vi "Test Threaded Parallel.vi"() -> ()   [LabVIEW 2021]
uses:
  Source/Support/Nodes/abs_Node/Status.ctl
  Test System/Test System.lvclass
  C:/Users/Tim/Documents/GitHub/LV_Behaviour_Tree/Source/System/bt_System.lvclass
  Source/Blackboard/Blackboard.lvclass
  Source/Support/Nodes/Decorators/Repeater/Support/Finish On - Type.ctl
  Source/Blackboard/Blackboard.lvclass/Blackboard.ctl
  Source/Support/Nodes/Leaves/abs_Type Leaf/abs_Type Leaf.lvclass/abs_Type Leaf.ctl
  Source/Support/Nodes/Composites/abs_Parallel/Support/Status Calculation.ctl
  Source/System/bt_System.lvclass/bt_System.ctl
  Source/Blackboard/Get Value Type/Get I32.vi
  <vilib>/TSA/Abstract Data Classes/Abs_Types/I32 Integer/Static Read.vi
  Source/System/Properties/Write Behaviour Tree.vi
  Source/Blackboard/Support/Index Group.vi
  Source/Blackboard/Support/Index Tags.vi
  Source/Support/Nodes/Leaves/abs_Type Leaf/Properties/Write Value Class.vi
  <vilib>/TSA/Omni-Bus/Local Bus/Support/I32/Local Bus_I32.lvclass
  C:/Program Files (x86)/National Instruments/LabVIEW 2021/vi.lib/TSA/Abstract Data Classes/Abs_Types/Value/Abs_Value.lvclass
  <vilib>/TSA/Abstract Data Classes/Abs_Types/I32 Integer/Abs_I32 Integer.lvclass
  C:/Program Files (x86)/National Instruments/LabVIEW 2021/vi.lib/TSA/Abstract Data Classes/Abs_Types/Numeric/Abs_Numeric.lvclass
  Source/Support/Nodes/Leaves/Test Boolean/Test Abs_Boolean.lvclass
  C:/Users/Tim/Documents/GitHub/LV_Behaviour_Tree/Source/Support/Nodes/abs_Node/bt_Node.lvclass
  C:/Users/Tim/Documents/GitHub/LV_Behaviour_Tree/BT Abstract Type/abs_Type Leaf/abs_Type Leaf.lvclass
  <vilib>/TSA/Abstract Data Classes/Abs_Types/Boolean/Abs_Boolean.lvclass
  C:/Program Files (x86)/National Instruments/LabVIEW 2021/vi.lib/TSA/Abstract Data Classes/Abs_Types/Type/Abs_Type.lvclass
  <vilib>/TSA/Omni-Bus/Local Bus/Support/Initialise DVR's.vi
  <vilib>/TSA/Abstract Data Classes/Functions/Math/Support/Increment/I32/Method.vi
  <vilib>/TSA/Abstract Data Classes/Constants/Support/I32/I32.vi
  <vilib>/TSA/Abstract Data Classes/Functions/Math/Support/Add/I32/Method.vi
  <vilib>/TSA/Abstract Data Classes/Functions/Compare/Support/Less/I32/Method.vi
  <vilib>/TSA/Abstract Data Classes/Abs_Types/Value/Abs_Value.lvclass
  <vilib>/TSA/Abstract Data Classes/Abs_Types/Type/Abs_Type.lvclass
  <vilib>/TSA/Omni-Bus/Local Bus/Support/DBL/Local Bus_DBL.lvclass
  <vilib>/TSA/Omni-Bus/Local Bus/Support/SGL/Local Bus_SGL.lvclass
  <vilib>/TSA/Omni-Bus/Local Bus/Support/EXT/Local Bus_EXT.lvclass
  <vilib>/TSA/Omni-Bus/Local Bus/Support/Bool/Local Bus_Boolean.lvclass
  <vilib>/TSA/Omni-Bus/Local Bus/Support/STR/Local Bus_String.lvclass
  <vilib>/TSA/Omni-Bus/Local Bus/Support/Variant/Local Bus_Variant.lvclass
  <vilib>/TSA/Omni-Bus/Local Bus/Support/WFM/Local Bus_Waveform.lvclass
  <vilib>/TSA/Omni-Bus/Local Bus/Support/Time/Local Bus_Time.lvclass
  <vilib>/TSA/Omni-Bus/Local Bus/Support/U8/Local Bus_U8.lvclass
  <vilib>/TSA/Omni-Bus/Local Bus/Support/U16/Local Bus_U16.lvclass
  <vilib>/TSA/Omni-Bus/Local Bus/Support/U32/Local Bus_U32.lvclass
  <vilib>/TSA/Omni-Bus/Local Bus/Support/U64/Local Bus_U64.lvclass
  <vilib>/TSA/Omni-Bus/Local Bus/Support/I8/Local Bus_I8.lvclass
  <vilib>/TSA/Omni-Bus/Local Bus/Support/I16/Local Bus_I16.lvclass
  <vilib>/TSA/Omni-Bus/Local Bus/Support/I64/Local Bus_I64.lvclass
  <vilib>/TSA/Omni-Bus/Local Bus/Support/CSGL/Local Bus_CSGL.lvclass
  <vilib>/TSA/Omni-Bus/Local Bus/Support/CDBL/Local Bus_CDBL.lvclass
  <vilib>/TSA/Omni-Bus/Local Bus/Support/CEXT/Local Bus_CEXT.lvclass
  Source/BT.lvlib
  Source/Support/Nodes/Decorators/Repeater/bt_Repeater.lvclass
  Source/System/bt_System.lvclass
  Source/Support/Nodes/Composites/abs_Parallel/bt_Parallel.lvclass
  C:/Program Files (x86)/National Instruments/LabVIEW 2021/vi.lib/TSA/Abstract Data Classes/Abs_Types/Integer/Abs_Integer.lvclass
  C:/Program Files (x86)/National Instruments/LabVIEW 2021/vi.lib/TSA/Abstract Data Classes/Abs_Types/I32 Integer/Abs_I32 Integer.lvclass
  Source/Support/Nodes/abs_Node/bt_Node.lvclass
  <vilib>/TSA/Abstract Data Classes/Constants/Support/I32/Const_I32.lvclass
  <vilib>/TSA/Abstract Data Classes/Functions/Compare/Support/Less/I32/Less_I32.lvclass
  <vilib>/TSA/Abstract Data Classes/Functions/Math/Support/Increment/I32/Increment_I32.lvclass
  <vilib>/TSA/Abstract Data Classes/Functions/Math/Support/Add/I32/Add_I32.lvclass
  C:/Users/Tim/Documents/GitHub/LV_Behaviour_Tree/Test/Test System/Test System.lvclass
panel:
  out "Finish Count":i32
  out "Count 2":i32
  out "Count 1":i32
  out "Status":T1
  in  "stop":bool
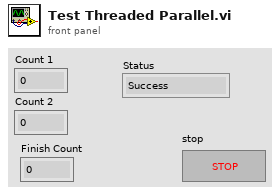
[diagram p1: front panel]
types:
  T1 = typedef "BT.lvlib/bt_Node.lvclass/Status.ctl" = enum16{"Success", "Failure", "Running"}
  T2 = typedef "BT.lvlib/bt_Repeater.lvclass/Finish On - Type.ctl" = enum16{"Success", "Failure", "Never"}
  T3 = typedef "Add_I32.lvclass/Abs_Type.ctl" = refnum<class "Abs_I32 Integer.lvclass">
  T4 = typedef "BT.lvlib/bt_Parallel.lvclass/Status Calculation.ctl" = enum16{"Succeed on All Succeed", "Failure on All Failure", "Succeed on Any Succeed", "Failure on Any Failure"}
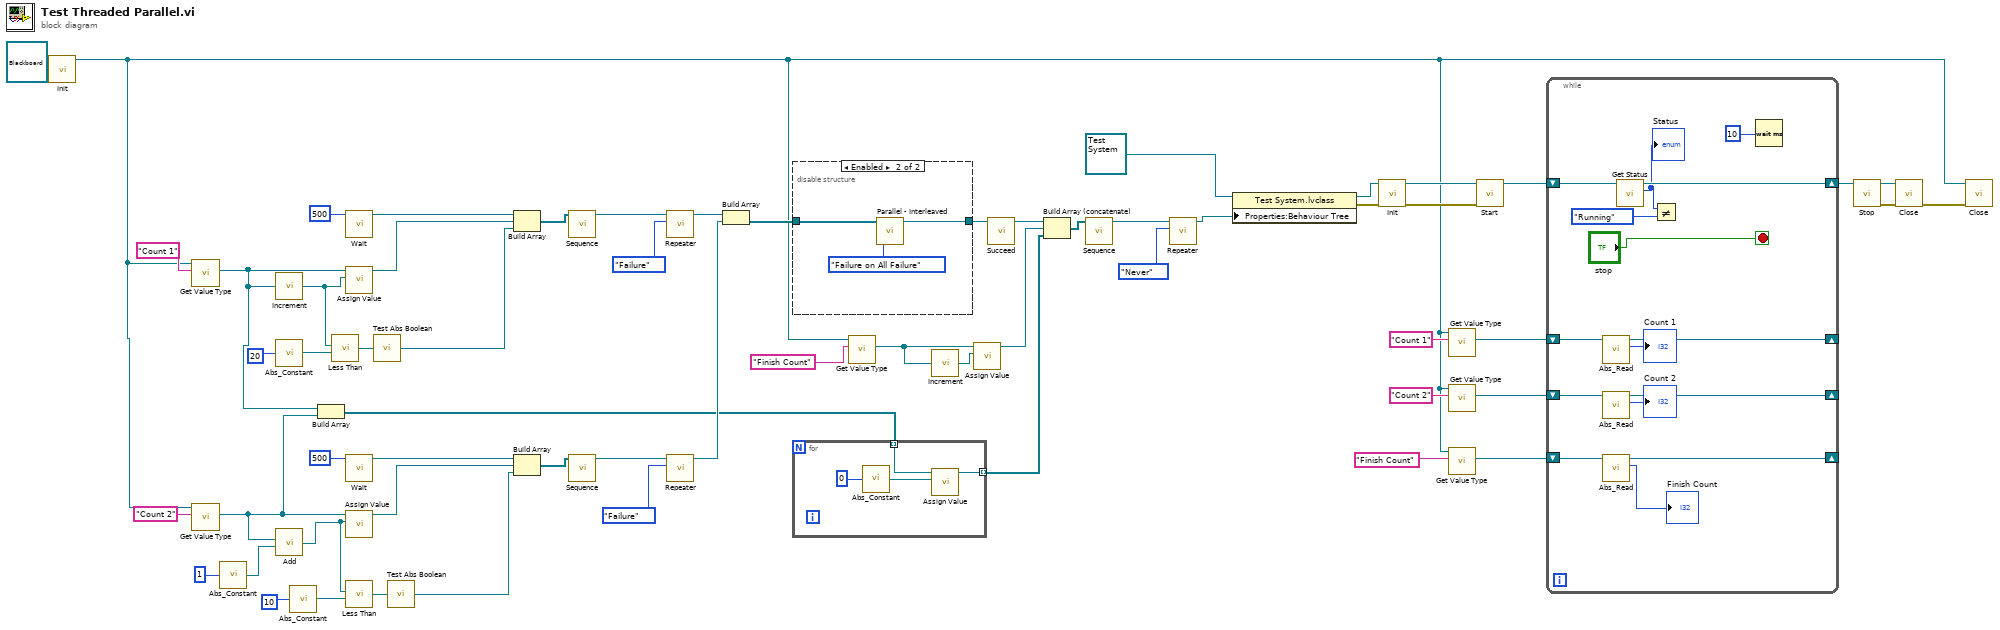
[diagram p0: block diagram]
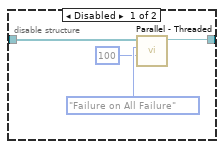
[diagram p2: hidden frame]
diagram:
  n1 = call-dynamic "Init.vi"("bt_Blackboard in"=refnum<class "Blackboard.lvclass"> refnum) -> ("bt_Blackboard out"=w10:refnum<class "Blackboard.lvclass">)  [unwired: 9 in, 1 out]
  n2 = call-poly "Get Value Type.vi"("Tag"="Count 1", "Blackboard in"=w10) -> ("Value"=w3:refnum<class "Abs_I32 Integer.lvclass">)  [unwired: 6 in, 3 out]
  n3 = call-poly "Get Value Type.vi"("Tag"="Count 2", "Blackboard in"=w10) -> ("Value"=w2:refnum<class "Abs_I32 Integer.lvclass">)  [unwired: 6 in, 3 out]
  n4 = call-poly <vilib>:"Abs_Constant.vi"("Value"=1) -> ("Constant"=w36:refnum<class "Abs_I32 Integer.lvclass">)  [unwired: 4 in]
  n5 = call-poly <vilib>:"Increment.vi"("Value"=w3) -> ("Result"=w21:refnum<class "Abs_I32 Integer.lvclass">)  [unwired: 4 in]
  n6 = call-poly <vilib>:"Abs_Constant.vi"("Value"=20) -> ("Constant"=w22:refnum<class "Abs_I32 Integer.lvclass">)  [unwired: 4 in]
  n7 = call-poly <vilib>:"Add.vi"("Input B"=w36, "Input A"=w2) -> ("Result"=w28:T3)  [unwired: 4 in]
  n8 = call-poly <vilib>:"Abs_Constant.vi"("Value"=10) -> ("Constant"=w27:refnum<class "Abs_I32 Integer.lvclass">)  [unwired: 4 in]
  n9 = Build Array(w3, w2) -> (w1:refnum<class "Abs_I32 Integer.lvclass">[])
  n10 = call-poly <vilib>:"Less Than.vi"("Value B"=w22, "Value A"=w21) -> ("Result"=w24:refnum<class "Abs_Boolean.lvclass">)  [unwired: 4 in]
  n11 = call "Wait.vi"("Time (ms)"=u32 500) -> ("Node Out"=w52:refnum<class "bt_Node.lvclass">)  [unwired: 10 in]
  n12 = call "Assign Value.vi"("Assigned Value"=w21, "Value"=w3) -> ("Node Out"=w46:refnum<class "bt_Node.lvclass">)  [unwired: 9 in]
  n13 = call "Wait.vi"("Time (ms)"=u32 500) -> ("Node Out"=w37:refnum<class "bt_Node.lvclass">)  [unwired: 10 in]
  n14 = call "Assign Value.vi"("Assigned Value"=w28, "Value"=w2) -> ("Node Out"=w40:refnum<class "bt_Node.lvclass">)  [unwired: 9 in]
  n15 = call-poly <vilib>:"Less Than.vi"("Value B"=w27, "Value A"=w28) -> ("Result"=w25:refnum<class "Abs_Boolean.lvclass">)  [unwired: 4 in]
  n16 = call "Test Abs Boolean.vi"("Abs_Boolean.lvclass"=w24) -> ("abs_Node"=w4:refnum<class "bt_Node.lvclass">)  [unwired: 4 in]
  n17 = call "Test Abs Boolean.vi"("Abs_Boolean.lvclass"=w25) -> ("abs_Node"=w6:refnum<class "bt_Node.lvclass">)  [unwired: 4 in]
  n18 = Build Array(w52, w46, w4) -> (w51:refnum<class "bt_Node.lvclass">[])
  n19 = Build Array(w37, w40, w6) -> (w38:refnum<class "bt_Node.lvclass">[])
  n20 = call "Sequence.vi"("Nodes"=w51) -> ("Node"=w34:refnum<class "bt_Node.lvclass">)  [unwired: 10 in]
  n21 = call "Sequence.vi"("Nodes"=w38) -> ("Node"=w30:refnum<class "bt_Node.lvclass">)  [unwired: 10 in]
  n22 = call "Repeater.vi"("Finish On"=Finish_On_-_Type."Failure", "Node In"=w34) -> ("Node Out"=w33:refnum<class "bt_Node.lvclass">)  [unwired: 9 in]
  n23 = call "Repeater.vi"("Finish On"=Finish_On_-_Type."Failure", "Node In"=w30) -> ("Node Out"=w29:refnum<class "bt_Node.lvclass">)  [unwired: 9 in]
  n24 = Build Array(w33, w29) -> (w20:refnum<class "bt_Node.lvclass">[])
  n25 = disable-structure shown="Enabled" {
    disable-tunnel: w20 -> [w64 w68]
    disable-tunnel: [w62 w67] -> w9
    frame Disabled {
      n26 = call "Parallel - Threaded.vi"("Test Interval (ms)"=100, "Status Calculation"=Status_Calculation."Failure on All Failure", "Nodes"=w64) -> ("Node"=w62:refnum<class "bt_Node.lvclass">)  [unwired: 8 in]
    }
    frame Enabled {
      n27 = call "Parallel - Interleaved.vi"("Status Calculation"=Status_Calculation."Failure on All Failure", "Nodes"=w68) -> ("Node"=w67:refnum<class "bt_Node.lvclass">)  [unwired: 9 in]
    }
  }
  n28 = for {
    tunnel: [w70] -> w5 mode=indexing
    tunnel: w1 -> [w69] mode=indexing
    n29 = call-poly <vilib>:"Abs_Constant.vi"("Value"=0) -> ("Constant"=w71:refnum<class "Abs_I32 Integer.lvclass">)  [unwired: 4 in]
    n30 = call "Assign Value.vi"("Assigned Value"=w71, "Value"=w69) -> ("Node Out"=w70:refnum<class "bt_Node.lvclass">)  [unwired: 9 in]
  }
  n31 = call-poly "Get Value Type.vi"("Tag"="Finish Count", "Blackboard in"=w10) -> ("Value"=w17:refnum<class "Abs_I32 Integer.lvclass">)  [unwired: 6 in, 3 out]
  n32 = call-poly <vilib>:"Increment.vi"("Value"=w17) -> ("Result"=w16:refnum<class "Abs_I32 Integer.lvclass">)  [unwired: 4 in]
  n33 = call "Assign Value.vi"("Assigned Value"=w16, "Value"=w17) -> ("Node Out"=w7:refnum<class "bt_Node.lvclass">)  [unwired: 9 in]
  n34 = call "Succeed.vi"("Node In"=w9) -> ("Node"=w8:refnum<class "bt_Node.lvclass">)  [unwired: 10 in]
  n35 = Build Array (concatenate)(w8, w7, w5) -> (w14:refnum<class "bt_Node.lvclass">[])
  n36 = call "Sequence.vi"("Nodes"=w14) -> ("Node"=w13:refnum<class "bt_Node.lvclass">)  [unwired: 10 in]
  n37 = call "Repeater.vi"("Finish On"=Finish_On_-_Type."Never", "Node In"=w13) -> ("Node Out"=w18:refnum<class "bt_Node.lvclass">)  [unwired: 9 in]
  n38 = property class="Test System.lvclass"(reference=refnum<class "Test System.lvclass"> refnum ("Test System.lvclass"), "Properties:Behaviour Tree"=w18) -> (reference out=w54:refnum<class "Test System.lvclass">, error out=w55:errorcluster)  [unwired: 1 in]
  n39 = call "Init.vi"("error in (no error)"=w55, "bt_System in"=w54) -> ("error out"=w60:errorcluster, "bt_System out"=w61:refnum<class "Test System.lvclass">)  [unwired: 8 in]
  n40 = call-poly "Get Value Type.vi"("Tag"="Count 1", "Blackboard in"=w10) -> ("Value"=w44:refnum<class "Abs_I32 Integer.lvclass">)  [unwired: 6 in, 3 out]
  n41 = call-poly "Get Value Type.vi"("Tag"="Count 2", "Blackboard in"=w10) -> ("Value"=w42:refnum<class "Abs_I32 Integer.lvclass">)  [unwired: 6 in, 3 out]
  n42 = call-poly "Get Value Type.vi"("Tag"="Finish Count", "Blackboard in"=w10) -> ("Value"=w12:refnum<class "Abs_I32 Integer.lvclass">)  [unwired: 6 in, 3 out]
  n43 = call "Start.vi"("error in (no error)"=w60, "bt_System in"=w61) -> ("bt_System out"=w59:refnum<class "Test System.lvclass">)  [unwired: 8 in, 1 out]
  n44 = while {
    shift-right: [w86] -> w58
    shift-left: w59 -> [w87]
    shift-right: [w83] -> _
    shift-left: w44 -> [w84]
    shift-right: [w81] -> _
    shift-left: w42 -> [w82]
    shift-right: [w73] -> _
    shift-left: w12 -> [w74]
    stop <- "stop" stop-if-true
    n45 = call-poly <vilib>:"Abs_Read.vi"("Abs_I32 Integer in"=w84) -> ("Value"=→"Count 1":i32, "Abs_I32 Integer out"=w83:refnum<class "Abs_I32 Integer.lvclass">)  [unwired: 8 in, 1 out]
    n46 = call-poly <vilib>:"Abs_Read.vi"("Abs_I32 Integer in"=w82) -> ("Value"=→"Count 2":i32, "Abs_I32 Integer out"=w81:refnum<class "Abs_I32 Integer.lvclass">)  [unwired: 8 in, 1 out]
    n47 = call-poly <vilib>:"Abs_Read.vi"("Abs_I32 Integer in"=w74) -> ("Value"=→"Finish Count":i32, "Abs_I32 Integer out"=w73:refnum<class "Abs_I32 Integer.lvclass">)  [unwired: 8 in, 1 out]
    n48 = call "Get Status.vi"("bt_System in"=w87) -> ("Status"=w78:T1, "bt_System out"=w86:refnum<class "Test System.lvclass">)  [unwired: 8 in, 1 out]
    "Status" <- w78
    n49 = Not Equal?(x=w78, y=Status."Running") -> ()  [unwired: 1 out]
    n50 = Wait (ms)(milliseconds to wait=u32 10) -> ()  [unwired: 1 out]
  }
  n51 = call "Stop.vi"("bt_System in"=w58) -> ("error out"=w56:errorcluster, "bt_System out"=w57:refnum<class "Test System.lvclass">)  [unwired: 9 in]
  n52 = call-dynamic "Close.vi"("error in (no error)"=w56, "bt_System in"=w57) -> ("error out"=w49:errorcluster)  [unwired: 8 in, 1 out]
  n53 = call-dynamic "Close.vi"("error in (no error)"=w49, "bt_Blackboard in"=w10) -> ()  [unwired: 8 in, 2 out]
